vi "getMDData.vi"(11 "MDILC in":refnum<class "MDILC.lvclass">) -> (2 "MDData":T1 {"Responses"."Displacement" items=["OK", "IllegalFunction", "IllegalDataAddress", "IllegalDataValue", "SlaveDeviceFailure", "Acknowledge", "SlaveDeviceBusy", "NegativeAcknowledge", "MemoryParityError", "GatewayPathUnavailable", "GatewayTargetDeviceFailedToRespond"]}, 3 "MDILC out":refnum<class "MDILC.lvclass">)   [LabVIEW 2016, in "RTMDILC.lvlib" / "MDILC.lvclass"]
uses:
  MDILC.lvclass
  DataTypes/MDData.ctl
  DataTypes/MDConstants.ctl
  DataTypes/MDTelemetry.ctl
  DataTypes/MDResponses.ctl
  Common_RT_Modbus/DataTypes/ExceptionCodes.ctl
  DataTypes/MDTimings.ctl
  MDILC.lvclass/MDILC.ctl
  RTMDILC.lvlib
  Common_RT_Modbus/RTModbus.lvlib
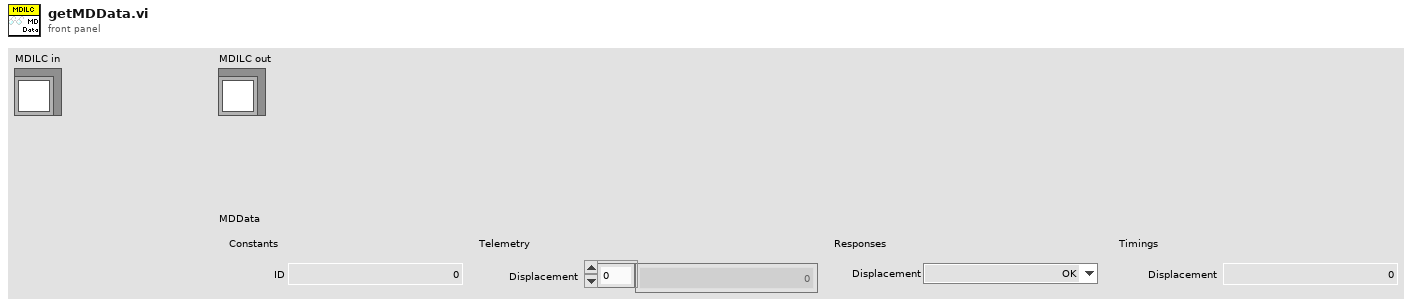
[diagram p1: front panel]
types:
  T1 = typedef "RTMDILC.lvlib/MDData.ctl" = cluster{"Constants":T2, "Telemetry":T3, "Responses":T4, "Timings":T6}
  T2 = typedef "RTMDILC.lvlib/MDConstants.ctl" = cluster{"ID":i16}
  T3 = typedef "RTMDILC.lvlib/MDTelemetry.ctl" = cluster{"Displacement":sgl[]}
  T4 = typedef "RTMDILC.lvlib/MDResponses.ctl" = cluster{"Displacement":T5}
  T5 = typedef "RTModbus.lvlib/ExceptionCodes.ctl" = u16
  T6 = typedef "RTMDILC.lvlib/MDTimings.ctl" = cluster{"Displacement":u32}
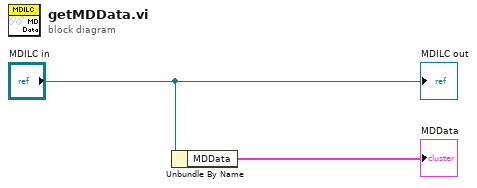
[diagram p0: block diagram]
diagram:
  n1 = Unbundle By Name("MDILC in") -> ("MDData"=→"MDData":T1)
  "MDILC out" <- "MDILC in"
